vi "Init_sequences.vi"(8 "error in (no error)":errorcluster, 11 "XML Elements":string) -> (0 "error IO":errorcluster, 3 "Sequences":T1(array[cluster]))   [LabVIEW 2016]
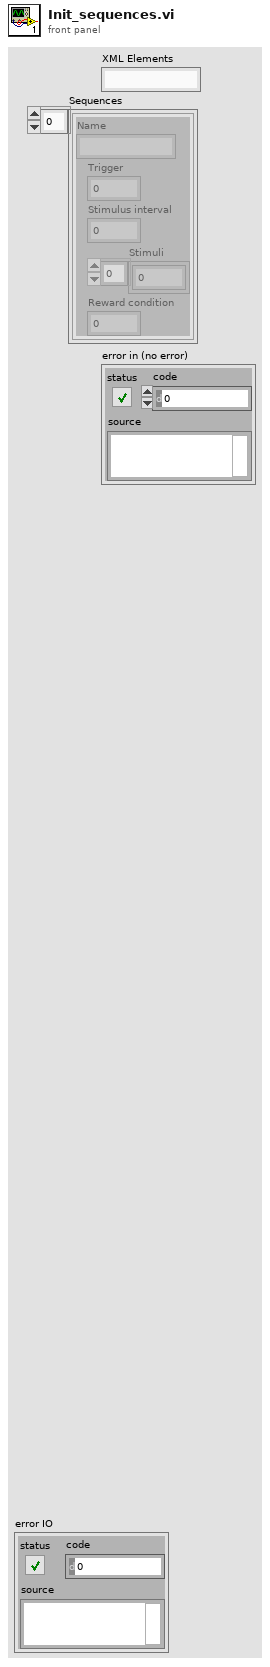
[diagram p1: front panel]
types:
  T1 = cluster{"Name":string, "Trigger":u16, "Stimulus interval":dbl, "Stimuli":i32[], "Reward condition":u16}[]
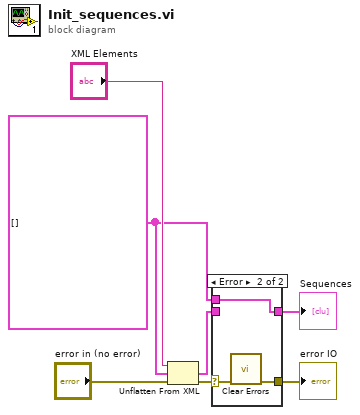
[diagram p0: block diagram]
diagram:
  w2 = T1 [] ("Sequences")
  n1 = Unflatten From XML(xml string="XML Elements", type=w2, error in (no error)="error in (no error)") -> (value=w3:T1, error out=w5:errorcluster)
  n2 = case shown="Error" w5 {
    selector: w5 -> [w9 w12]
    tunnel: [w9 w11] -> w4
    tunnel: [w8 w10] -> w1
    tunnel: w3 -> [w8 _]
    tunnel: w2 -> [_ w10]
    frame No Error {
    }
    frame Error {
      n3 = call <vilib>:"Clear Errors.vi"("error in (no error)"=w12) -> ("error out"=w11:errorcluster)  [unwired: 5 in, 1 out]
    }
  }
  "error IO" <- w4
  "Sequences" <- w1
